vi "Set Enable Debugging.vi"(8 "error in (no error)":errorcluster, 9 "Wait for debugger on launch (false)":bool, 10 "Enable debugging (false)":bool, 11 "NI_AB_API_Targetfile in":refnum<class "NI_AB_API_Targetfile.lvclass">) -> (0 "error out":errorcluster, 3 "NI_AB_API_Targetfile out":refnum<class "NI_AB_API_Targetfile.lvclass">)   [LabVIEW 2020, in "NI_AB_API_Targetfile.lvclass"]
uses:
  <vilib>/AppBuilder/AB_API/Targetfile/NI_AB_API_Targetfile.lvclass
  e:/builds/penguin/labview/branches/2020/dev/dist/vi.lib/AppBuilder/AB_API/Build/NI_AB_API_Build.lvclass
  <vilib>/AppBuilder/AB_Classes/TargetFile/AB_Targetfile.lvclass
  e:/builds/penguin/labview/branches/2020/dev/dist/vi.lib/AppBuilder/AB_Classes/Build/AB_Build.lvclass
  <vilib>/AppBuilder/AB_API/Targetfile/NI_AB_API_Targetfile.lvclass/NI_AB_API_Targetfile.ctl
  <vilib>/AppBuilder/AB_API/Build/NI_AB_API_Build.lvclass
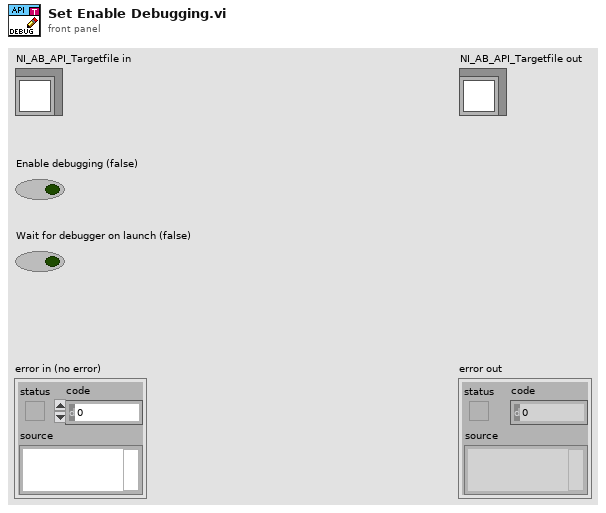
[diagram p1: front panel]
types:
  T1 = typedef "AB_Targetfile.ctl" = cluster{"targetfileName":string, "targetfileGUID":string, "enableDebugging":bool, "versionInfo":cluster{"productName":string, "legalCopyright":string, "companyName":string, "internalName":string, "fileDescription":string}, "eng_consolidatedTypeInfo":string, "fastFileFormat":bool, "eng_LEIFBuildData":u32, "versionIndependent":bool}
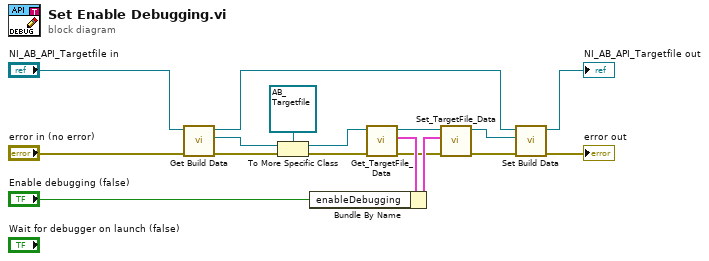
[diagram p0: block diagram]
diagram:
  n1 = call <vilib>:"Get Build Data.vi"("error in (no error)"="error in (no error)", "NI_AB_API_Build in"="NI_AB_API_Targetfile in") -> ("error out"=w5:errorcluster, "AB_Build.lvclass"=w7:refnum<class "AB_Build.lvclass">, "NI_AB_API_Build out"=w9:refnum<class "NI_AB_API_Targetfile.lvclass">)  [unwired: 7 in]
  n2 = To More Specific Class(target class=refnum<class "AB_Targetfile.lvclass"> refnum ("AB_Targetfile in"), reference=w7, error in=w5) -> (specific class reference=w6:refnum<class "AB_Targetfile.lvclass">, error out=w3:errorcluster)
  n3 = call <vilib>:"Get_TargetFile_Data.vi"("error in (no error)"=w3, "AB_Targetfile in"=w6) -> ("error out"=w2:errorcluster, "data"=w11:T1, "AB_Targetfile out"=w12:refnum<class "AB_Targetfile.lvclass">)  [unwired: 7 in]
  n4 = Bundle By Name(cluster=w11, "enableDebugging"="Enable debugging (false)") -> (w10:T1)
  n5 = call <vilib>:"Set_TargetFile_Data.vi"("error in (no error)"=w2, "data"=w10, "AB_Targetfile in"=w12) -> ("error out"=w1:errorcluster, "AB_Targetfile out"=w4:refnum<class "AB_Targetfile.lvclass">)  [unwired: 7 in]
  n6 = call <vilib>:"Set Build Data.vi"("error in (no error)"=w1, "AB_Build.lvclass"=w4, "NI_AB_API_Build in"=w9) -> ("error out"=→"error out":errorcluster, "NI_AB_API_Build out"=→"NI_AB_API_Targetfile out":refnum<class "NI_AB_API_Targetfile.lvclass">)  [unwired: 7 in]
